vi "ADCP_read_packet_from_serial_port.vi"(0 "ADCP In":refnum<class "ADCP.lvclass">, 11 "error in (no error)":errorcluster) -> (1 "Checksum Valid ?":bool, 2 "Packet Type":T1(ring), 3 "Packet_Priority":enum16{"LOW", "HIGH"}(ring), 4 "ADCP out":refnum<class "ADCP.lvclass">, 6 "Received Packet":u8[](array[numeric]), 8 "Packet node ID":u8, 10 "Packet frame ID":u8, 15 "error out":errorcluster)   [LabVIEW 2017, in "ADCP.lvclass"]
uses:
  ADCP.lvclass
  ADCP.lvclass/ADCP.ctl
  <vilib>/Instr/_visa.llb/VISA Flush IO Buffer Mask.ctl
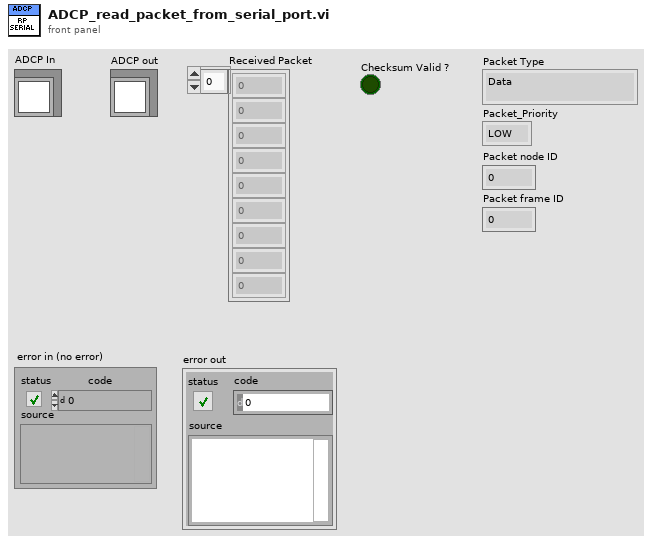
[diagram p1: front panel]
types:
  T1 = enum16{"Data", "Connection Management", "Remote Request", "Error and status", "INVALID"}
  T2 = typedef "VISA Flush IO Buffer Mask.ctl" = u16
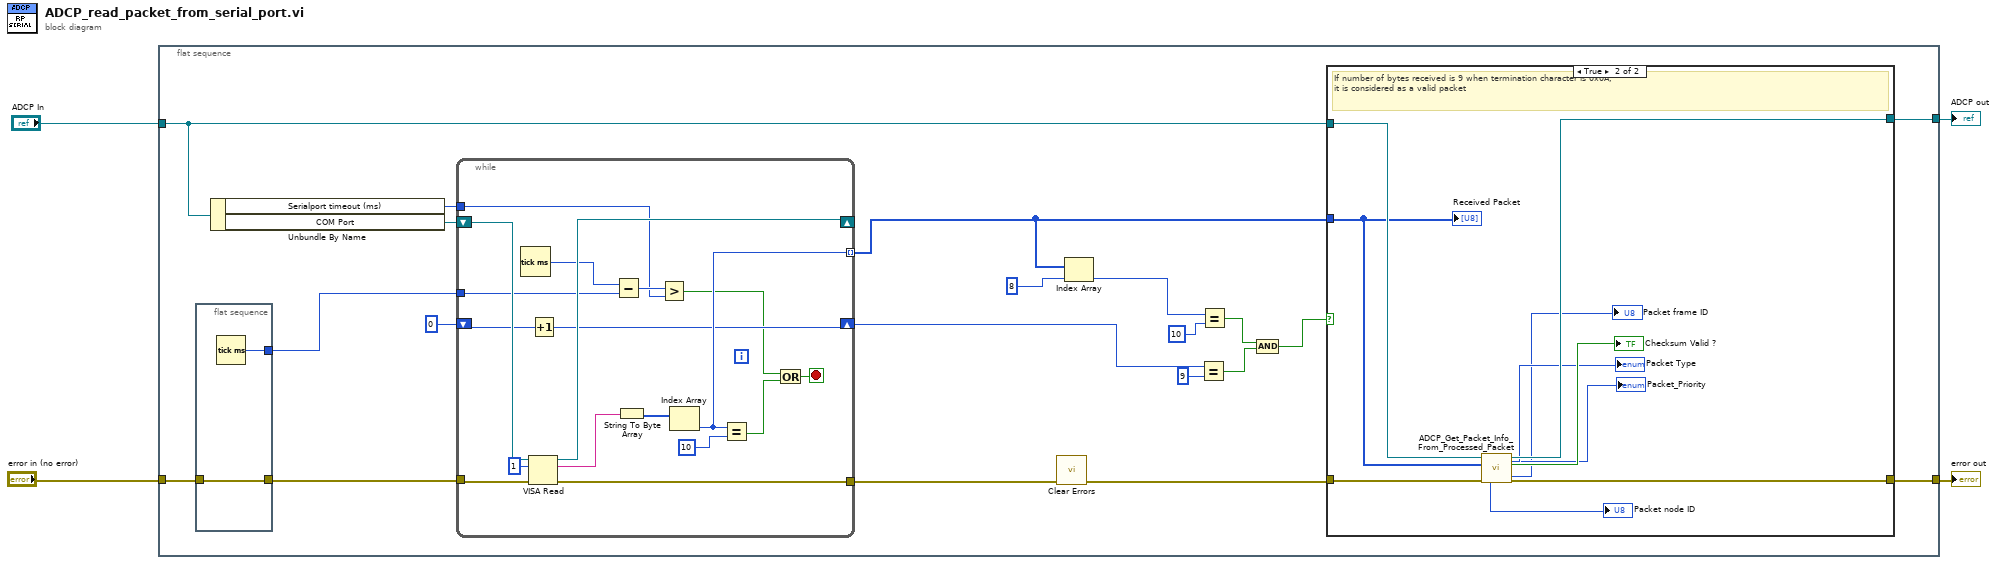
[diagram p0: block diagram]
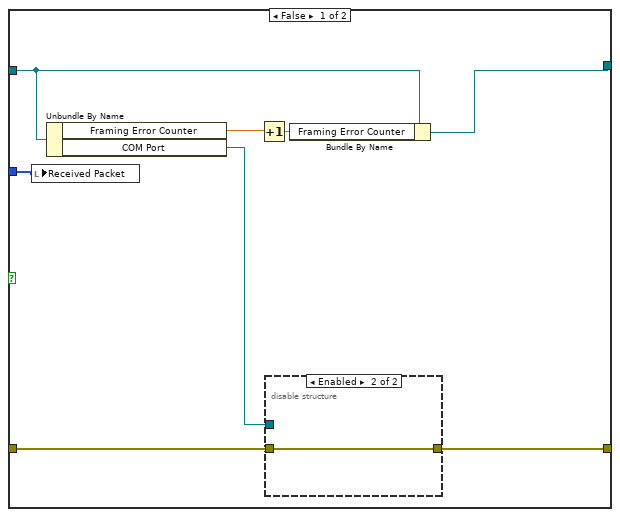
[diagram p2: hidden frame]
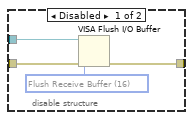
[diagram p3: hidden frame]
diagram:
  n1 = flat-sequence {
    tunnel: "ADCP In" -> [w21]
    tunnel: "error in (no error)" -> [w24]
    tunnel: [w22] -> w2
    tunnel: [w20] -> w1
    frame #0 {
      n2 = flat-sequence {
        tunnel: w24 -> [w67]
        tunnel: [w67] -> w17
        tunnel: [w66] -> w8
        frame #0 {
          n3 = Tick Count (ms)() -> (millisecond timer value=w66:u32)
        }
      }
      n4 = Unbundle By Name(w21) -> ("Serialport timeout (ms)"=w7:u32, "COM Port"=w16:refnum<visa-resource-name>)
      n5 = while {
        tunnel: w17 -> [w42]
        shift-right: [w40] -> _
        shift-left: w16 -> [w41]
        tunnel: [w35] -> w15 mode=indexing
        tunnel: [w34] -> w6
        shift-right: [w32] -> w12
        shift-left: 0 -> [w33]
        tunnel: w8 -> [w30]
        tunnel: w7 -> [w28]
        stop <- w27 stop-if-true
        n6 = Tick Count (ms)() -> (millisecond timer value=w31:u32)
        n7 = VISA Read(VISA resource name=w41, byte count=u32 1, error in (no error)=w42) -> (VISA resource name out=w40:refnum<visa-resource-name>, read buffer=w38:string, error out=w34:errorcluster)  [unwired: 1 out]
        n8 = Increment(x=w33) -> (x+1=w32:i32)
        n9 = Subtract(x=w31, y=w30) -> (x-y=w29:u32)
        n10 = String To Byte Array(string=w38) -> (unsigned byte array=w37:u8[])
        n11 = Greater?(x=w29, y=w28) -> (0:w25:bool)
        n12 = Index Array(array=w37) -> (element=w35:u8)  [unwired: 1 in]
        n13 = Equal?(x=w35, y=u8 10) -> (x = y?=w26:bool)
        n14 = Or(x=w25, y=w26) -> (x .or. y?=w27:bool)
      }
      n15 = call <vilib>:"Clear Errors.vi"("error in (no error)"=w6) -> ("error out"=w5:errorcluster)  [unwired: 5 in, 1 out]
      n16 = Index Array(array=w15, index=8) -> (element=w18:u8)
      n17 = Equal?(x=w12, y=9) -> (x = y?=w11:bool)
      n18 = Equal?(x=w18, y=10) -> (x = y?=w14:bool)
      n19 = And(x=w14, y=w11) -> (x .and. y?=w9:bool)
      n20 = case shown="True" w9 {
        tunnel: w5 -> [w45 w65]
        tunnel: w15 -> [w46 w62]
        tunnel: [w44 w64] -> w22
        tunnel: w21 -> [w48 w63]
        tunnel: [w47 w61] -> w20
        frame False {
          n21 = local write "Received Packet"(w46) -> ()
          n22 = Unbundle By Name(w48) -> ("Framing Error Counter"=w50:dbl, "COM Port"=w43:refnum<visa-resource-name>)
          n23 = Increment(x=w50) -> (x+1=w49:dbl)
          n24 = disable-structure shown="Enabled" {
            disable-tunnel: w45 -> [w54 w55]
            disable-tunnel: [w53 w55] -> w44
            disable-tunnel: w43 -> [w52 _]
            frame Disabled {
              w51 = T2 16 items=["Flush Receive Buffer"=16, "Write Transmit Buffer to Device"=32, "Flush Receive Buffer (No I/O)"=64, "Flush Transmit Buffer"=128] ("Mask")
              n25 = VISA Flush I/O Buffer(VISA resource name=w52, mask (16)=w51, error in (no error)=w54) -> (error out=w53:errorcluster)  [unwired: 1 out]
            }
            frame Enabled {
            }
          }
          n26 = Bundle By Name(cluster=w48, "Framing Error Counter"=w49) -> (w47:refnum<class "ADCP.lvclass">)
        }
        frame True {
          # "If number of bytes received is 9 when termination character is 0x0A,\nit is considered as a valid packet"
          n27 = call "ADCP_Get_Packet_Info_From_Processed_Packet.vi"("error in (no error)"=w65, "Processed Packet"=w62, "ADCP in"=w63) -> ("error out"=w64:errorcluster, "Checksum Valid ?"=→"Checksum Valid ?":bool, "ADCP out"=w61:refnum<class "ADCP.lvclass">, "Packet frame ID"=→"Packet frame ID":u8, "Packet Type"=→"Packet Type":T1, "Packet node ID"=→"Packet node ID":u8, "Packet_Priority"=→"Packet_Priority":enum16{"LOW", "HIGH"})  [unwired: 2 in]
          "Received Packet" <- w62
        }
      }
    }
  }
  "error out" <- w2
  "ADCP out" <- w1
